vi "ifr2025 Sinad Setup  .vi"(8 "error in (no error)":errorcluster {"code" format="%.0x"}, 11 "instrument handle":refnum<visa-resource-name>) -> (0 "error out":errorcluster {"code" format="%.0x"}, 1 "Filter Weighting":i16, 2 "Averages":i16, 3 "instrument handle out":refnum<visa-resource-name>, 4 "Mode":i16, 5 "Target Sinad":dbl, 6 "Delta Level Step":dbl)   [LabVIEW 2009]
doc: "This VI returns parameter values relating to the Sinad measurement system."
uses:
  Ifr2025_32.dll
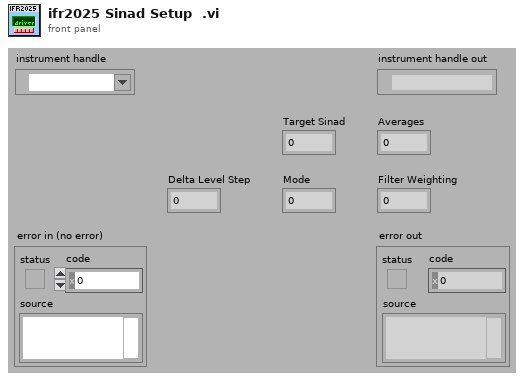
[diagram p1: front panel]
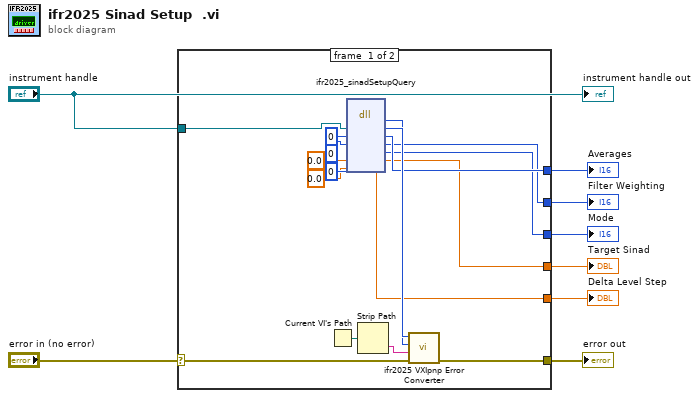
[diagram p0: block diagram]
diagram:
  n1 = case shown="No Error" "error in (no error)" {
    selector: "error in (no error)" -> [w20 w26]
    tunnel: [w19 w26] -> w8
    tunnel: "instrument handle" -> [w24 _]
    tunnel: [w17 _] -> w5
    tunnel: [w15 _] -> w4
    tunnel: [w13 _] -> w3
    tunnel: [w11 _] -> w2
    tunnel: [w9 _] -> w1
    frame #0 {
      n2 = Current VI's Path() -> (path=w25:path)
      n3 = dll-call lib="P:/inst/Marconi 2024 Signal Generator/source/labview/ifr2025/ifr2025/ifr2025_*.*" fn="ifr2025_sinadSetupQuery"("vi"=w24, "Averages"=i16 0, "Filter Weighting"=i16 0, "Mode"=i16 0, "Target Sinad"=0.0, "Delta Level Step"=0.0) -> (w22:i32, "vi"=w23:u32, "Averages"=w17:i16, "Filter Weighting"=w15:i16, "Mode"=w13:i16, "Target Sinad"=w11:dbl, "Delta Level Step"=w9:dbl)  [unwired: 3 in, 2 out]
      n4 = Strip Path(path=w25) -> (name=w21:string)  [unwired: 1 out]
      n5 = call "ifr2025 VXIpnp Error Converter.vi"("error in (no error)"=w20, "name of VI (\"\")"=w21, "CVI error code (0)"=w22, "instrument handle"=w23) -> ("error out"=w19:errorcluster)  [unwired: 7 out]
    }
    frame #1 {
    }
  }
  "error out" <- w8
  "Averages" <- w5
  "Filter Weighting" <- w4
  "Mode" <- w3
  "Target Sinad" <- w2
  "Delta Level Step" <- w1
  "instrument handle out" <- "instrument handle"
